vi "Poll.vi"(8 "error in (no error)":errorcluster, 11 "PLC in":refnum<class "MB PLC Client.lvclass">) -> (0 "error out":errorcluster, 3 "PLC out":refnum<class "MB PLC Client.lvclass">)   [LabVIEW 2018, in "MB PLC Client.lvlib" / "MB PLC Client.lvclass"]
uses:
  MB PLC Client.lvclass
  MB PLC Client.lvclass/MB PLC Client.ctl
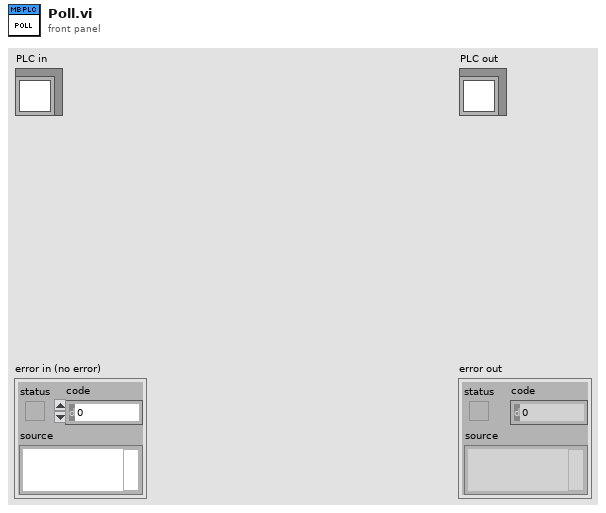
[diagram p1: front panel]
types:
  T1 = typedef "MB PLC Client.lvlib/MB Ref Range_Cluster.ctl" = cluster{"Start":u32, "Qty":u16}
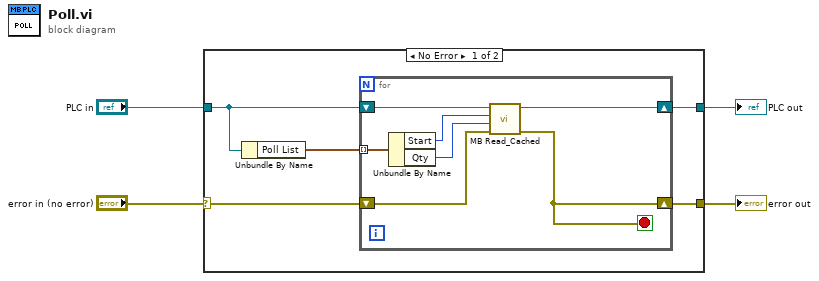
[diagram p0: block diagram]
diagram:
  n1 = case shown="No Error" "error in (no error)" {
    selector: "error in (no error)" -> [w6 w17]
    tunnel: "PLC in" -> [w9 w18]
    tunnel: [w7 w18] -> w2
    tunnel: [w5 w17] -> w1
    frame No Error {
      n2 = Unbundle By Name(w9) -> ("Poll List"=w8:T1[])
      n3 = for {
        shift-right: [w15] -> w7
        shift-left: w9 -> [w16]
        tunnel: w8 -> [w14] mode=indexing
        shift-right: [w10] -> w5
        shift-left: w6 -> [w11]
        stop <- w10 stop-if-true
        n4 = Unbundle By Name(w14) -> ("Start"=w13:u32, "Qty"=w12:u16)
        n5 = call "MB Read_Cached.vi"("error in (no error)"=w11, "Quantity(1)"=w12, "Modbus Reference"=w13, "MB PLC in"=w16) -> ("error out"=w10:errorcluster, "MB PLC out"=w15:refnum<class "MB PLC Client.lvclass">)  [unwired: 6 in]
      }
    }
    frame Error {
    }
  }
  "error out" <- w1
  "PLC out" <- w2
